vi "Vision Processing.vi"(4 "error in (no error)":errorcluster) -> ()   [LabVIEW 2013]
doc: "This VI runs in parallel to other tasks. It gets images from the camera, processes them for color or shape and use that information to affect robot behavior."
uses:
  <vilib>/Rock Robotics/WPI/Camera/WPI_CameraImageSize.ctl
  Vision/TargetType.ctl
  Robot Global Data.vi
panel:
  in  "y":bool
  in  "Score Limit 2":dbl=80.0
  in  "Image Size 2":T1=enum."320x240"
  in  "Color Components 2":T2={"Hue"={108.0, 140.0}, "Sat"={97.0, 255.0}, "Val"={178.0, 255.0}} {"Val" scale=0.0..255.0; "Sat" scale=0.0..255.0; "Hue" scale=0.0..255.0 scale format="%#_3g"}
  out "Hot 2":bool
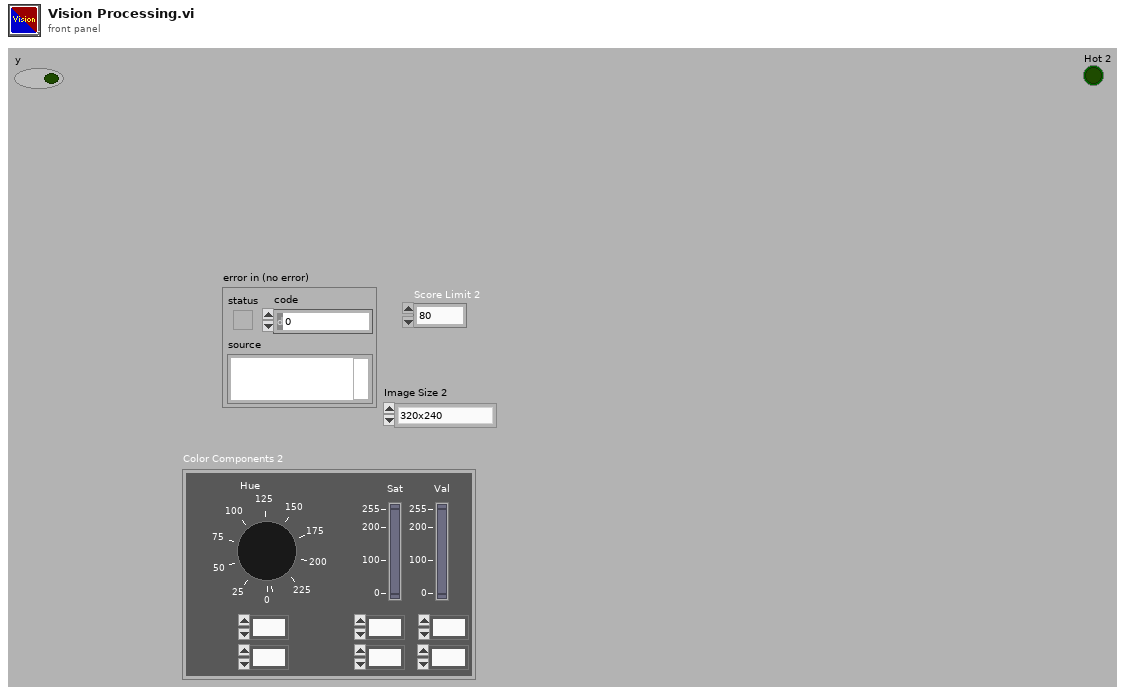
[diagram p1: front panel]
types:
  T1 = typedef "WPI_CameraImageSize.ctl" = enum16{"640x480", "320x240", "160x120"}
  T2 = cluster{"Hue":cluster{dbl, dbl}, "Sat":cluster{dbl, dbl}, "Val":cluster{dbl, dbl}}
  T3 = typedef "Image Type" = u32
  T4 = typedef "WPI_CameraDevRef.ctl" = cluster{"Camera Address":string, "CameraStatus":errorcluster, "Acquire Image Notifier":refnum<notifier>}
  T5 = typedef "IMAQ Image.ctl" = refnum<image>
  T6 = typedef "TargetType.ctl" = enum16{"Not Hot", "Hot"}
  T7 = cluster{"Horizontal":bool, "Aspect Score":dbl, "Rect Score":dbl, cluster{"Left":dbl, "Top":dbl, "Right":dbl, "Bottom":dbl}, "Equiv H":dbl, "Equiv V":dbl}[]
  T8 = cluster{"Scores":cluster{"Total":dbl, "Left":dbl, "Right":dbl, "Ratio":dbl, "Vertical":dbl, "index":i32, "State":T6}, "Verticals":cluster{"Horizontal?":bool, "Aspect Score":dbl, "Rect Score":dbl, cluster{"Left":dbl, "Top":dbl, "Right":dbl, "Bottom":dbl}, "Equiv H":dbl, "Equiv V":dbl}, "Horizontals":cluster{"Horizontal?":bool, "Aspect Score":dbl, "Rect Score":dbl, cluster{"Left":dbl, "Top":dbl, "Right":dbl, "Bottom":dbl}, "Equiv H":dbl, "Equiv V":dbl}, "Validated":bool}[]
  T9 = cluster{"Scores":cluster{"Total":dbl, "Left":dbl, "Right":dbl, "Ratio":dbl, "Vertical":dbl, "index":i32, "State":T6}, "Verticals":cluster{"Horizontal?":bool, "Aspect Score":dbl, "Rect Score":dbl, cluster{"Left":dbl, "Top":dbl, "Right":dbl, "Bottom":dbl}, "Equiv H":dbl, "Equiv V":dbl}, "Horizontals":cluster{"Horizontal?":bool, "Aspect Score":dbl, "Rect Score":dbl, cluster{"Left":dbl, "Top":dbl, "Right":dbl, "Bottom":dbl}, "Equiv H":dbl, "Equiv V":dbl}, "Validated":bool}
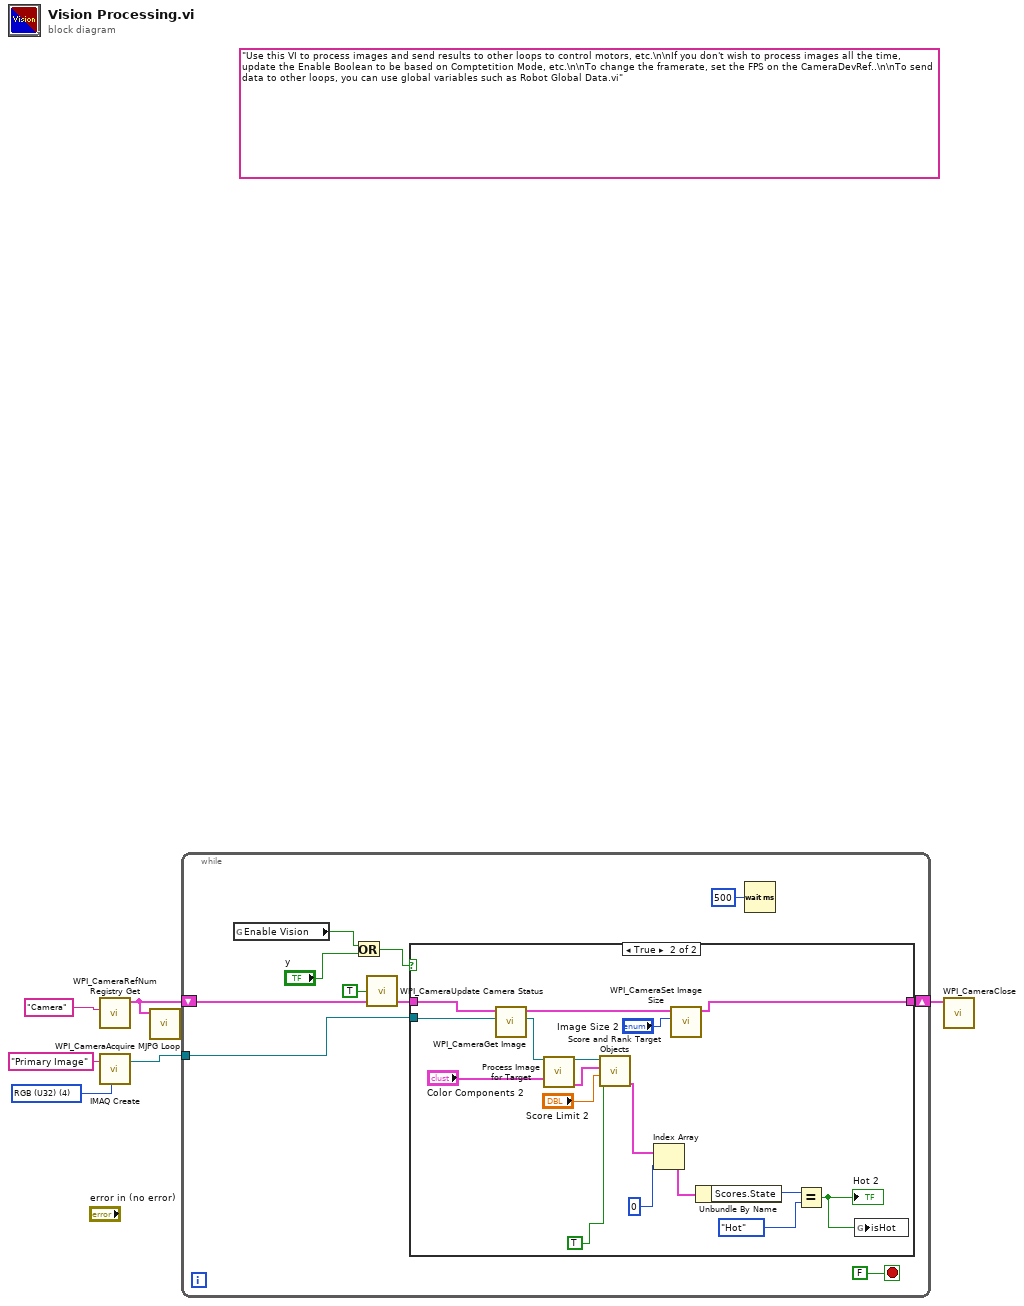
[diagram p0: block diagram]
diagram:
  w6 = T3 4 items=["Grayscale (U8)", "Grayscale (I16)", "Grayscale (SGL)", "Complex (CSG)", "RGB (U32)", "HSL (U32)", "RGB (U64)"] ("Image Type")
  (unwired) "Use this VI to process images and send results to other loops to control motors, etc.\n\nIf you don't wish to process images all the time, update the Enable Boolean to be based on Comptetition Mode, etc.\n\nTo change the framerate, set the FPS on the CameraDevRef..\n\nTo send data to other loops, you can use global variables such as Robot Global Data.vi"
  n1 = call <vilib>:"WPI_CameraRefNum Registry Get.vi"("refnum name"="Camera") -> ("CameraDevRef"=w2:T4)  [unwired: 9 in, 1 out]
  n2 = call "IMAQ Create"("Image Name"="Primary Image", "Image Type"=w6) -> ("New Image"=w4:T5)  [unwired: 2 in, 2 out]
  n3 = call <vilib>:"WPI_CameraAcquire MJPG Loop.vi"("CameraDevRef"=w2) -> ()  [unwired: 11 in]
  n4 = while {
    tunnel: w4 -> [w16]
    shift-right: [w15] -> w3
    shift-left: w2 -> [w14]
    stop <- FALSE stop-if-true
    n5 = global read "Robot Global Data.vi" "Enable Vision"() -> (w9:bool)
    n6 = Or(x=w9, y="y") -> (x .or. y?=w7:bool)
    n7 = call <vilib>:"WPI_CameraUpdate Camera Status.vi"("CameraDevRef In"=w14, "Enable Vision"=TRUE) -> ("CameraDevRef Out"=w13:T4)  [unwired: 3 in]
    n8 = case shown="True" w7 {
      tunnel: w16 -> [_ w33]
      tunnel: [w17 w34] -> w15
      tunnel: w13 -> [w17 w32]
      frame False {
      }
      frame True {
        n9 = call <vilib>:"WPI_CameraGet Image.vi"("Image"=w33, "CameraDevRef"=w32) -> ("Image Out"=w30:T5, "CameraDevRef Out"=w31:T4)  [unwired: 1 in, 7 out]
        n10 = call "Process Image for Target.vi"("Src Image"=w30, "Color Components"="Color Components 2") -> ("Src Image Out"=w29:T5, "Particles"=w28:T7)  [unwired: 11 in, 1 out]
        n11 = call "Score and Rank Target Objects.vi"("Annotate"=TRUE, "Score Limit"="Score Limit 2", "Particles"=w28, "Image in"=w29) -> ("Target Info"=w24:T8)  [unwired: 6 in, 1 out]
        n12 = Index Array(array=w24, index=0) -> (element=w22:T9)
        n13 = call <vilib>:"WPI_CameraSet Image Size.vi"("Image Size"="Image Size 2", "CameraDevRef"=w31) -> ("CameraDevRef Out"=w34:T4)  [unwired: 1 in, 8 out]
        n14 = Unbundle By Name(w22) -> ("Scores.State"=w21:T6)
        n15 = Equal?(x=w21, y=TargetType."Hot" ("Scores.State")) -> (x = y?=w19:bool)
        "Hot 2" <- w19
        n16 = global write "Robot Global Data.vi" "isHot"(w19) -> ()
      }
    }
    n17 = Wait (ms)(milliseconds to wait=u32 500) -> ()  [unwired: 1 out]
  }
  n18 = call <vilib>:"WPI_CameraClose.vi"("CameraDevRef"=w3) -> ()  [unwired: 1 in, 10 out]
